vi "delta_k.vi"(9 "t_k":dbl, 10 "O_k":dbl) -> (2 "delta_k":dbl)   [LabVIEW 2014]
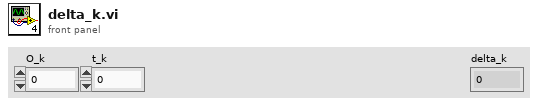
[diagram p1: front panel]
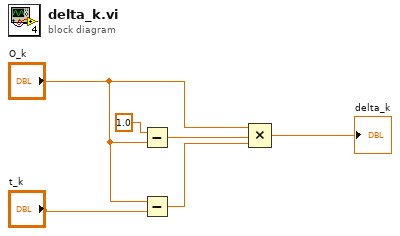
[diagram p0: block diagram]
diagram:
  n1 = Subtract(x=1.0, y="O_k") -> (x-y=w4:dbl)
  n2 = Subtract(x="O_k", y="t_k") -> (x-y=w1:dbl)
  n3 = Compound Arithmetic op=MULTIPLY("O_k", w4, w1) -> (→"delta_k":dbl)
